vi "ExtWndEvents.vi"(8 "ErrI":errorcluster) -> (0 "ErrO":errorcluster)   [LabVIEW 2016]
panel:
  out "Other Parameters":sgl[](array[numeric]) format="%.2f"
  out "Coordinates":i32[](array[numeric])
  out "Tool":i32(ring) items=["Point", "Line", "Rectangle", "Oval", "Polygon", "Freehand Region", "Annulus", "Rotated Rectangle", "Zoom", "Pan", "Broken Line", "Freehand Line"]
  out "Event":i32(ring) items=["No  event", "Click event", "Draw event", "Move event", "Size event", "Scroll event", "Activate event", "Close event", "Double click event"]
  in  "stop":bool
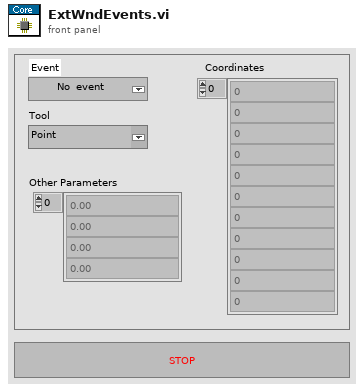
[diagram p1: front panel]
types:
  T1 = typedef "Image Type" = u32
  T2 = typedef "IMAQ Image.ctl" = refnum<image>
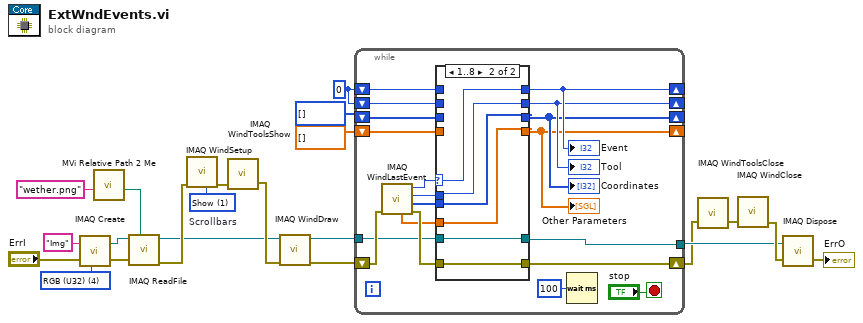
[diagram p0: block diagram]
diagram:
  w10 = 0 ("Event")
  w22 = T1 4 items=["Grayscale (U8)", "Grayscale (I16)", "Grayscale (SGL)", "Complex (CSG)", "RGB (U32)", "HSL (U32)", "RGB (U64)", "Grayscale (U16)"] ("Image Type")
  w21 = 1 items=["Hide", "Show", "No change"]  # Scrollbars
  n1 = call "IMAQ Create"("Image Name"="Img", "Image Type"=w22, "error in (no error)"="ErrI") -> ("New Image"=w20:T2, "error out"=w18:errorcluster)  [unwired: 2 in]
  n2 = call "MVi Relative Path 2 Me.vi"("Relative Path"="wether.png") -> ("Appended Dir"=w1:path)  [unwired: 5 in, 1 out]
  n3 = call "IMAQ ReadFile"("File Path"=w1, "error in (no error)"=w18, "Image"=w20) -> ("error out"=w19:errorcluster, "Image Out"=w4:T2)  [unwired: 4 in, 3 out]
  n4 = call "IMAQ WindSetup"("Scrollbars (No change)"=w21, "error in (no error)"=w19) -> ("error out"=w6:errorcluster)  [unwired: 9 in]
  n5 = call "IMAQ WindToolsShow"("error in (no error)"=w6) -> ("error out"=w5:errorcluster)  [unwired: 4 in, 1 out]
  n6 = call "IMAQ WindDraw"("error in (no error)"=w5, "Image"=w4) -> ("error out"=w3:errorcluster, "Image Out (duplicate)"=w14:T2)  [unwired: 8 in]
  n7 = while "ExtWndEventhandler::by Gaoke Yang (gaoke.yang@yahoo.com)" {
    shift-right: [w37] -> w8
    shift-left: w3 -> [w41]
    tunnel: w14 -> [w28]
    tunnel: [w27] -> w12
    shift-right: [w26] -> _
    shift-left: w10 -> [w32]
    shift-right: [w25] -> _
    shift-left: w10 -> [w31]
    shift-right: [w24] -> _
    shift-left: i32[] [] ("Coordinates") -> [w30]
    shift-right: [w23] -> _
    shift-left: sgl[] [] ("Other Parameters") -> [w29]
    stop <- "stop" stop-if-true
    n8 = call "IMAQ WindLastEvent"("error in (no error)"=w41) -> ("error out"=w38:errorcluster, "Coordinates"=w34:i32[], "Tool"=w35:i32, "Event"=w36:i32, "Other Parameters"=w33:sgl[])  [unwired: 5 in, 1 out]
    n9 = case shown="1..8" w36 {
      selector: w36 -> [_ w52]
      tunnel: w38 -> [w42 w53]
      tunnel: [w42 w53] -> w37
      tunnel: w35 -> [_ w51]
      tunnel: w34 -> [_ w50]
      tunnel: w33 -> [_ w49]
      tunnel: [w47 w52] -> w26
      tunnel: [w46 w51] -> w25
      tunnel: [w45 w50] -> w24
      tunnel: [w44 w49] -> w23
      tunnel: w32 -> [w47 _]
      tunnel: w31 -> [w46 _]
      tunnel: w30 -> [w45 _]
      tunnel: w29 -> [w44 _]
      tunnel: w28 -> [w43 w48]
      tunnel: [w43 w48] -> w27
      frame 0, Default {
      }
      frame 1..8 {
      }
    }
    "Event" <- w26
    "Tool" <- w25
    "Coordinates" <- w24
    "Other Parameters" <- w23
    n10 = Wait (ms)(milliseconds to wait=u32 100) -> ()  [unwired: 1 out]
  }
  n11 = call "IMAQ WindToolsClose"("error in (no error)"=w8) -> ("error out"=w7:errorcluster)  [unwired: 5 in]
  n12 = call "IMAQ WindClose"("error in (no error)"=w7) -> ("error out"=w13:errorcluster)  [unwired: 5 in]
  n13 = call "IMAQ Dispose"("Image"=w12, "error in (no error)"=w13) -> ("error out"=→"ErrO":errorcluster)  [unwired: 4 in]
